vi "Clase5a.vi"() -> ()   [LabVIEW 2011]
panel:
  in  "Seleccionador local":u16(ring) items=["Local 1", "Local 2", "Local 3"]
  out "A/C":bool
  out "NumeroPersonas":i32
  out "Temperatura":i32(slide) scale=0.0..100.0
  # "Debemos seleccionar el local, luego generar el nuero de personas entre 1-50 y la temperatura\nentre 1-60.\nEl A/C se enciende de acuerdo a los siguientes casos:\n\nLocal   condicion para encender el A/C\nLocal 1 Si la temperatura es mayor a 25 o el numero de empleados es mayor a 30\nLocal 2 Si la temperatura es mayor a 28 o el numero de empleados es mayor a 35\nLocal 3 Si la temperatura es mayor a 24 o el numero de empleados es mayor a 20"
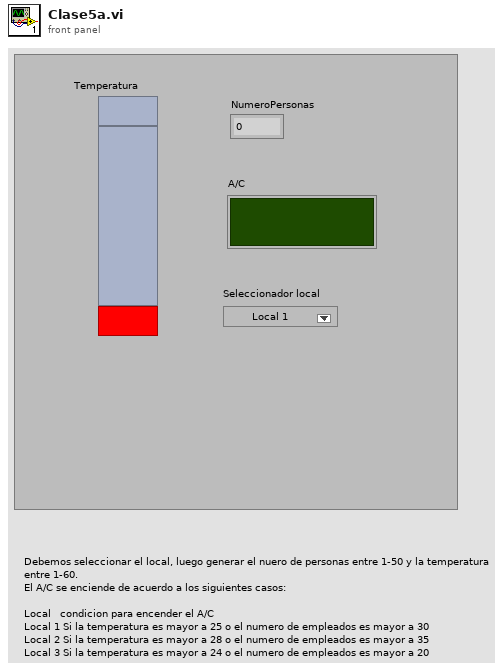
[diagram p1: front panel]
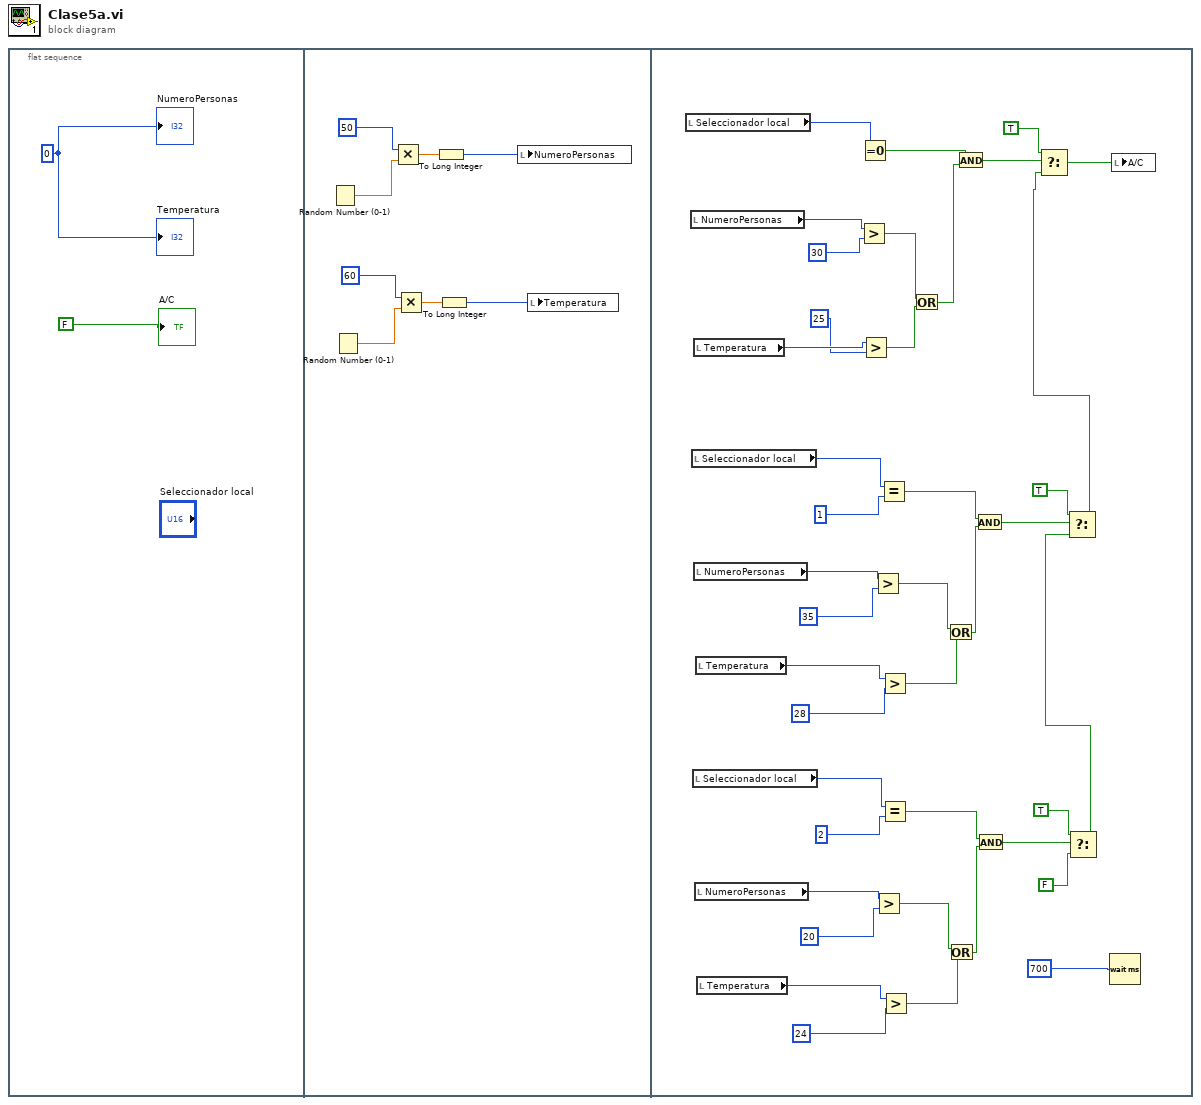
[diagram p0: block diagram]
diagram:
  n1 = flat-sequence {
    frame #0 {
      w1 = 0
      "Temperatura" <- w1
      "NumeroPersonas" <- w1
      "A/C" <- FALSE
    }
    frame #1 {
      n2 = Random Number (0-1)() -> (number: 0 to 1=w9:dbl)
      n3 = Random Number (0-1)() -> (number: 0 to 1=w6:dbl)
      n4 = Multiply(x=50, y=w9) -> (x*y=w8:dbl)
      n5 = Multiply(x=60, y=w6) -> (x*y=w4:dbl)
      n6 = To Long Integer(number=w8) -> (32bit integer=w7:i32)
      n7 = To Long Integer(number=w4) -> (32bit integer=w3:i32)
      n8 = local write "NumeroPersonas"(w7) -> ()
      n9 = local write "Temperatura"(w3) -> ()
    }
    frame #2 {
      n10 = local read "Seleccionador local"() -> (w50:u16)
      n11 = local read "NumeroPersonas"() -> (w49:i32)
      n12 = local read "Seleccionador local"() -> (w38:u16)
      n13 = local read "Seleccionador local"() -> (w14:u16)
      n14 = local read "Temperatura"() -> (w46:i32)
      n15 = local read "NumeroPersonas"() -> (w36:i32)
      n16 = local read "NumeroPersonas"() -> (w16:i32)
      n17 = local read "Temperatura"() -> (w34:i32)
      n18 = local read "Temperatura"() -> (w18:i32)
      n19 = Greater?(x=w49, y=30) -> (0:w47:bool)
      n20 = Equal To 0?(x=w50) -> (x = 0?=w43:bool)
      n21 = Greater?(x=w46, y=25) -> (0:w44:bool)
      n22 = Greater?(x=w36, y=35) -> (0:w32:bool)
      n23 = Greater?(x=w16, y=20) -> (0:w20:bool)
      n24 = Equal?(x=w38, y=1) -> (x = y?=w30:bool)
      n25 = Greater?(x=w34, y=28) -> (0:w31:bool)
      n26 = Equal?(x=w14, y=2) -> (x = y?=w22:bool)
      n27 = Greater?(x=w18, y=24) -> (0:w21:bool)
      n28 = Or(x=w47, y=w44) -> (x .or. y?=w42:bool)
      n29 = Or(x=w32, y=w31) -> (x .or. y?=w29:bool)
      n30 = Or(x=w20, y=w21) -> (x .or. y?=w23:bool)
      n31 = And(x=w43, y=w42) -> (x .and. y?=w41:bool)
      n32 = And(x=w30, y=w29) -> (x .and. y?=w27:bool)
      n33 = And(x=w22, y=w23) -> (x .and. y?=w25:bool)
      n34 = Select(t=TRUE, s=w25, f=FALSE) -> (s? t:f=w13:bool)
      n35 = Select(t=TRUE, s=w27, f=w13) -> (s? t:f=w26:bool)
      n36 = Select(t=TRUE, s=w41, f=w26) -> (s? t:f=w39:bool)
      n37 = Wait (ms)(milliseconds to wait=700) -> ()  [unwired: 1 out]
      n38 = local write "A/C"(w39) -> ()
    }
  }
